vi "get_sharedVariable.vi"(8 "error in (no error)":errorcluster, 11 "HGF_SVVarManVisitor_create in":refnum<class "HGF_SVVarManVisitor_create.lvclass">) -> (0 "error out":errorcluster, 2 "shared variable":refnum<k21>, 3 "HGF_SVVarManVisitor_create out":refnum<class "HGF_SVVarManVisitor_create.lvclass">)   [LabVIEW 2012, in "HGF_SV.lvlib" / "HGF_SVVarManVisitor_create.lvclass"]
uses:
  HGF_SVVarManVisitor_create.lvclass
  HGF_SVVarManVisitor_create.lvclass/HGF_SVVarManVisitor_create.ctl
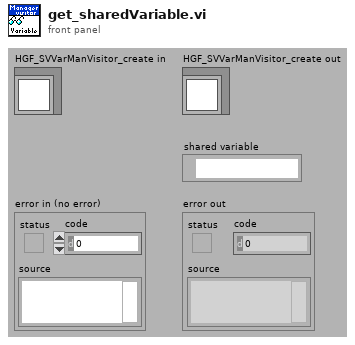
[diagram p1: front panel]
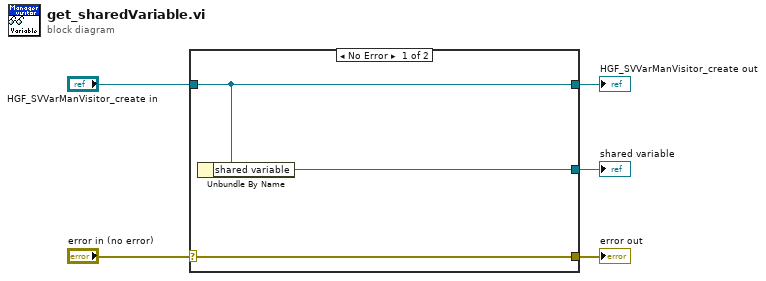
[diagram p0: block diagram]
diagram:
  n1 = case shown="No Error" "error in (no error)" {
    selector: "error in (no error)" -> [w8 w9]
    tunnel: [w8 w9] -> w4
    tunnel: [w7 w10] -> w2
    tunnel: "HGF_SVVarManVisitor_create in" -> [w7 w10]
    tunnel: [w6 _] -> w1
    frame No Error {
      n2 = Unbundle By Name(w7) -> ("shared variable"=w6:refnum<k21>)
    }
    frame Error {
    }
  }
  "error out" <- w4
  "HGF_SVVarManVisitor_create out" <- w2
  "shared variable" <- w1
